vi "Perform Step.vi"(8 "error in (no error)":errorcluster, 11 "Numeric Assertion in":refnum<class "Numeric Assertion.lvclass">) -> (0 "error out":errorcluster, 2 "Result":T1, 3 "Numeric Assertion out":refnum<class "Numeric Assertion.lvclass">)   [LabVIEW 2020, in "MacroAssert.lvlib" / "Numeric Assertion.lvclass"]
uses:
  Numeric Assertion.lvclass
  Numeric Assertion.lvclass/Numeric Assertion.ctl
  MacroAssert.lvlib
  CTLs/Report Data.ctl
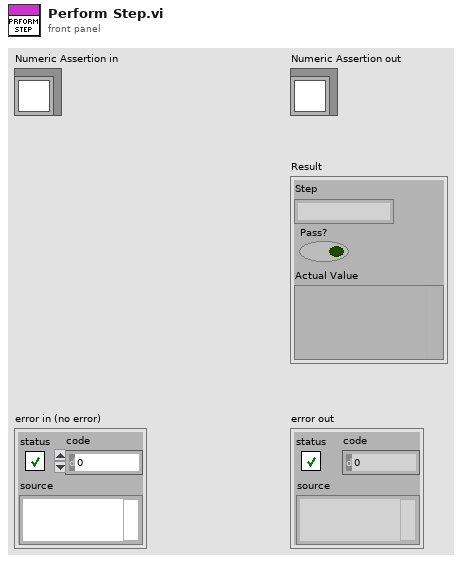
[diagram p1: front panel]
types:
  T1 = typedef "MacroAssert.lvlib/Report Data.ctl" = cluster{"Step":string, "Pass?":bool, "Actual Value":variant}
  T2 = enum8{"Enabled", "Disabled", "Disabled and Grayed Out"}
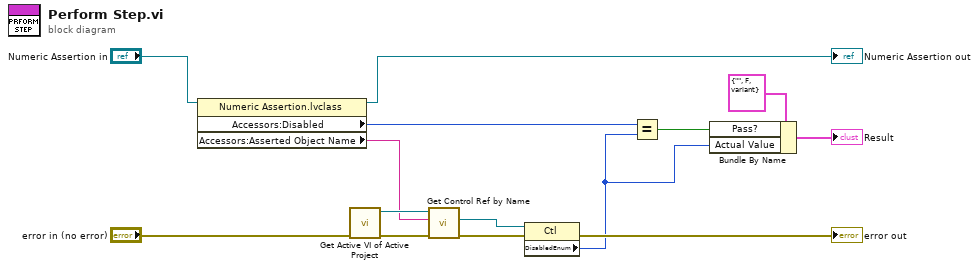
[diagram p0: block diagram]
diagram:
  n1 = property class="Numeric Assertion.lvclass"(reference="Numeric Assertion in") -> (reference out=→"Numeric Assertion out":refnum<class "Numeric Assertion.lvclass">, "Accessors:Disabled"=w8:T2, "Accessors:Asserted Object Name"=w9:string)  [unwired: 1 in, 1 out]
  n2 = call "Get Active VI of Active Project.vi"("error in (no error)"="error in (no error)") -> ("error out"=w14:errorcluster, "Active VI Ref"=w13:refnum<vi>)  [unwired: 9 in]
  n3 = call "Get Control Ref by Name.vi"("error in (no error)"=w14, "Name"=w9, "VI Ref"=w13) -> ("error out"=w4:errorcluster, "Ctl Ref"=w3:refnum<vi>)  [unwired: 6 in, 1 out]
  n4 = property class="Ctl"(reference=w3, error in=w4) -> (error out=→"error out":errorcluster, "DisabledEnum"=w1:T2)  [unwired: 1 out]
  n5 = Equal?(x=w8, y=w1) -> (x = y?=w6:bool)
  n6 = Bundle By Name(cluster=T1 {"Step"="", "Pass?"=FALSE, "Actual Value"=variant} ("Report Data"), "Pass?"=w6, "Actual Value"=w1) -> (→"Result":T1)
